vi "getInputGain.vi"(8 "error in (no error)":errorcluster, 11 "Instrument.LockinAPI in":refnum<class "Instrument.LockinAPI.lvclass">) -> (0 "error out":errorcluster, 2 "InputGain":dbl[](array[numeric]), 3 "Instrument.LockinAPI out":refnum<class "Instrument.LockinAPI.lvclass">)   [LabVIEW 2019, in "Instrument.LockinAPI.lvclass"]
doc: "API to get the AI waveforms.\n\nIf address=\"\", this API reads from localhost\nIf address is remote lockin, you need to add this computer to allowed whitelist on the lockin computer you are trying to access."
uses:
  Instrument.LockinAPI.lvclass
  C:/Users/patrick/Documents/GitHub/Instrument-Framework/lvsrc/Instrument/Instrument.lvclass
  Typedefs/API/LockinAPI.Commands--Enum.ctl
  ff94430c-509d-422d-b830-2f7b8ce5f6e0.vi
  ff94430c-509d-422d-b830-2f7b8ce5f6e0.vi/6f69bc81-23ec-4ebf-9497-0a50895ef104.vi
  ff94430c-509d-422d-b830-2f7b8ce5f6e0.vi/6f69bc81-23ec-4ebf-9497-0a50895ef104.vi/2cfbe149-ef36-44a5-8801-bc722fe13a4a.vi
  ff94430c-509d-422d-b830-2f7b8ce5f6e0.vi/6f69bc81-23ec-4ebf-9497-0a50895ef104.vi/60986b03-3f40-4761-9a5b-ff0a5eead437.vi
  ff94430c-509d-422d-b830-2f7b8ce5f6e0.vi/6f69bc81-23ec-4ebf-9497-0a50895ef104.vi/7a08f783-14c7-44aa-b280-33a9790b1e4a.vi
  <vilib>/JDP Science/JSONtext/Make JSON Array.vi
  ff94430c-509d-422d-b830-2f7b8ce5f6e0.vi/6f69bc81-23ec-4ebf-9497-0a50895ef104.vi/60986b03-3f40-4761-9a5b-ff0a5eead437.vi/71d2c03e-252d-415d-b3ec-da27a2405835.vi
  ff94430c-509d-422d-b830-2f7b8ce5f6e0.vi/6f69bc81-23ec-4ebf-9497-0a50895ef104.vi/7a08f783-14c7-44aa-b280-33a9790b1e4a.vi/44f7e792-1154-44e1-a42a-731c36b02aae.vi
  ff94430c-509d-422d-b830-2f7b8ce5f6e0.vi/6f69bc81-23ec-4ebf-9497-0a50895ef104.vi/7a08f783-14c7-44aa-b280-33a9790b1e4a.vi/58448f93-14b5-4f8f-a307-ab141e45290b.vi
  Instrument/API/Enum to String.vi
  Instrument/Private/Get RC Connection Status.vi
  <vilib>/JDP Science/JSONtext/Variant to JSON Text.vi
  <vilib>/JDP Science/JSONtext/support/Format JSON Array Text.vi
  Instrument/API/Send and Receive.vi
  <vilib>/JDP Science/JSONtext/JSON text to Variant.vi
  <vilib>/Utility/Data Type/Get Type Information.vi
  <vilib>/JDP Science/JSONtext/LVClass Serializer/JSONtext LVClass Serializer.lvclass
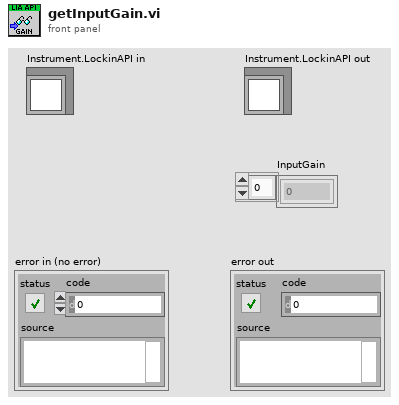
[diagram p1: front panel]
types:
  T1 = typedef "Instrument.LockinAPI.lvclass/LockinAPI.Commands--Enum.ctl" = enum16{"setAI", "setAO", "setAO_Amplitude", "setAO_DC", "setAO_Frequency", "setAO_Phase", "setAO_Function", "setAO_I+", "setREF", "setREF_Frequency", "setREF_Phase", "setREF_TC", "setREF_Roll-Off", "setDAQ", "setSampling", "setOffset", "setState", "getState", "getAO", "getAI", "getResults", "getSampling", "getAOconfig", "getREFconfig", "setInputGain", "setOutputGain", "getInputGain", "getOutputGain", "setSamplingMode", "getSamplingMode", "setSweep", "setSweepTime", "setSweepTable", "getStatus", "getSweepResults", "getSweepWaveforms", "startSweep", "stopSweep", "setAUX", "getAUX"}
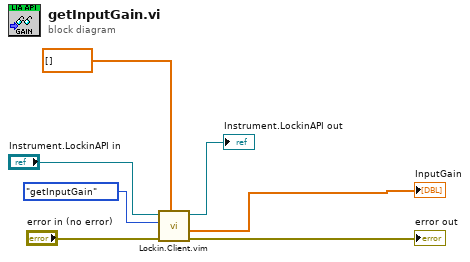
[diagram p0: block diagram]
diagram:
  n1 = call "Lockin.Client.vim"("Data Out type"=dbl[] [] ("InputGain"), "error in (no error)"="error in (no error)", "Command"=LockinAPI.Commands--Enum."getInputGain", "Instrument.LockinAPI in"="Instrument.LockinAPI in") -> ("error out"=→"error out":errorcluster, "Data out"=→"InputGain":dbl[], "Instrument.LockinAPI out"=→"Instrument.LockinAPI out":refnum<class "Instrument.LockinAPI.lvclass">)  [unwired: 5 in]
